vi "SetM1DefaultAccel.vi"(0 "VISA Refnum in":refnum<visa-resource-name>, 1 "Accel":u32, 2 "Address":u8, 3 "error in (no error)":errorcluster, 4 "Deccel":u32) -> (5 "VISA Refnum out":refnum<visa-resource-name>, 6 "Valid":bool, 7 "error out":errorcluster)   [LabVIEW 2015, in "Ion Motion Roboclaw.lvlib"]
uses:
  <instrlib>/Ion Motion Roboclaw/Ion Motion Roboclaw.lvlib
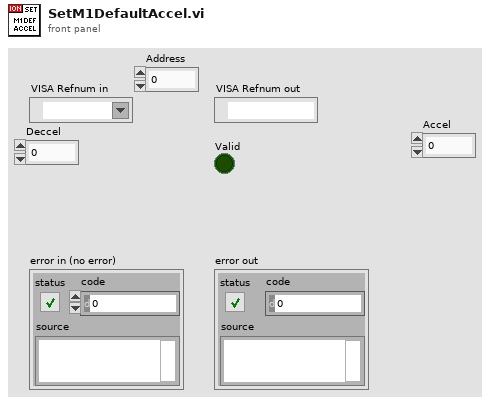
[diagram p1: front panel]
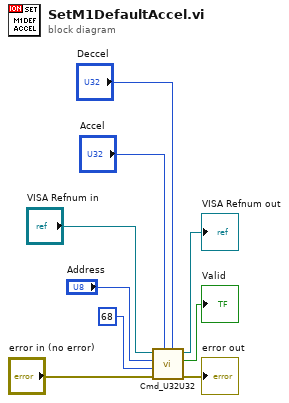
[diagram p0: block diagram]
diagram:
  n1 = call <instrlib>:"Cmd_U32U32.vi"("Arg2"="Deccel", "Arg1"="Accel", "error in (no error)"="error in (no error)", "Cmd"=u8 68, "Address"="Address", "VISA Refnum in"="VISA Refnum in") -> ("error out"=→"error out":errorcluster, "Valid"=→"Valid":bool, "VISA Refnum out"=→"VISA Refnum out":refnum<visa-resource-name>)  [unwired: 3 in]
